vi "NEW Test Step Parser.vi"(0 "CMD Cluster IN":T1, 5 "Controller?":bool, 7 "Profile":string[][](array[string]), 11 "Step":i32) -> (4 "CMD Cluster Out":T1, 8 "Time":dbl, 15 "Speed":bool)   [LabVIEW 2013]
uses:
  TypeDef/Command Cluster.ctl
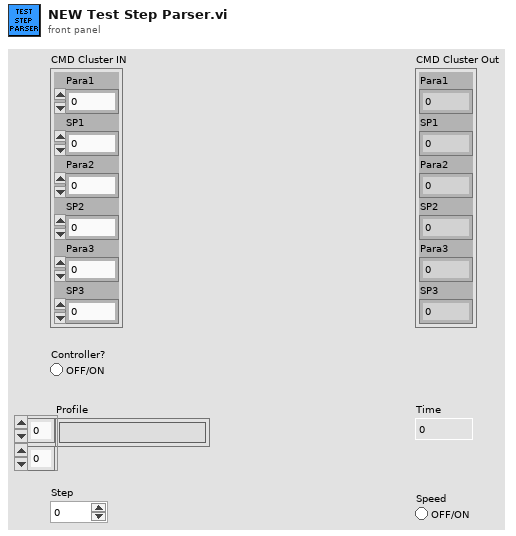
[diagram p1: front panel]
types:
  T1 = typedef "Command Cluster.ctl" = cluster{"Para1":i32, "SP1":dbl, "Para2":i32, "SP2":dbl, "Para3":i32, "SP3":dbl}
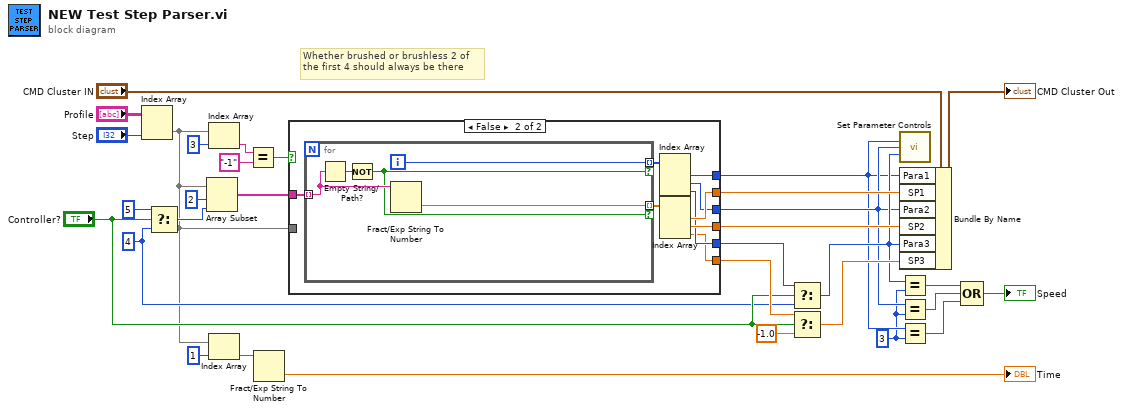
[diagram p0: block diagram]
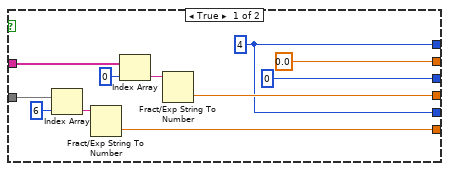
[diagram p2: hidden frame]
diagram:
  w6 = 3 ("y")
  w14 = 4 ("index")
  # "Whether brushed or brushless 2 of\nthe first 4 should always be there"
  n1 = Index Array(array="Profile", index (col)="Step") -> (element=w4:string[])  [unwired: 1 in]
  n2 = Select(t=5 ("length"), s="Controller?", f=w14) -> (s? t:f=w19:i32)
  n3 = Array Subset(array=w4, index=2, length=w19) -> (w27:string[])
  n4 = Index Array(array=w4, index=3) -> (element=w23:string)
  n5 = Index Array(array=w4, index=1) -> (element=w2:string)
  n6 = Equal?(x=w23, y="-1") -> (x = y?=w21:bool)
  n7 = Fract/Exp String To Number(string=w2) -> (number=→"Time":dbl)  [unwired: 3 in, 1 out]
  n8 = case shown="False" w21 {
    tunnel: w27 -> [w43 w52]
    tunnel: [0.0 w49] -> w26
    tunnel: [w40 w48] -> w25
    tunnel: [w37 w47] -> w7
    tunnel: [0 w46] -> w11
    tunnel: [w37 w45] -> w16
    tunnel: [w33 w44] -> w18
    tunnel: w4 -> [w34 _]
    frame True {
      w37 = 4
      n9 = Index Array(array=w34, index=6) -> (element=w35:string)
      n10 = Fract/Exp String To Number(string=w35) -> (number=w33:dbl)  [unwired: 3 in, 1 out]
      n11 = Index Array(array=w43, index=0) -> (element=w41:string)
      n12 = Fract/Exp String To Number(string=w41) -> (number=w40:dbl)  [unwired: 3 in, 1 out]
    }
    frame False {
      n13 = for {
        tunnel: w52 -> [w57] mode=indexing
        tunnel: [w53] -> w51 mode=indexing if=w54
        tunnel: [w55] -> w50 mode=indexing if=w54
        i -> [w55]
        n14 = Empty String/Path?(string/path=w57) -> (empty?=w56:bool)
        n15 = Not(x=w56) -> (.not. x?=w54:bool)
        n16 = Fract/Exp String To Number(string=w57) -> (number=w53:dbl)  [unwired: 3 in, 1 out]
      }
      n17 = Index Array(array=w50) -> (element #1=w47:i32, element #2=w46:i32, element #3=w45:i32)  [unwired: 3 in]
      n18 = Index Array(array=w51) -> (element #1=w49:dbl, element #2=w48:dbl, element #3=w44:dbl)  [unwired: 3 in]
    }
  }
  n19 = Select(t=w16, s="Controller?", f=w14) -> (s? t:f=w12:i32)
  n20 = Select(t=w18, s="Controller?", f=-1.0) -> (s? t:f=w15:dbl)
  n21 = call "Set Parameter Controls.vi"("Para 1"=w7, "Para 2"=w11, "Para 3"=w12) -> ()  [unwired: 12 in, 1 out]
  n22 = Bundle By Name(cluster="CMD Cluster IN", "Para1"=w7, "SP1"=w26, "Para2"=w11, "SP2"=w25, "Para3"=w12, "SP3"=w15) -> (→"CMD Cluster Out":T1)
  n23 = Equal?(x=w12, y=w6) -> (x = y?=w10:bool)
  n24 = Equal?(x=w11, y=w6) -> (x = y?=w9:bool)
  n25 = Equal?(x=w7, y=w6) -> (x = y?=w8:bool)
  n26 = Compound Arithmetic op=OR(w10, w9, w8) -> (→"Speed":bool)
